vi "DFD Kaiser Order Estimation.vi"(6 "fs [Hz]":dbl=1.0 format="%.2f", 7 "filter type":T3(ring), 8 "error in (no error)":errorcluster, 9 "order option":enum16{"MinNum", "MinEven", "MinOdd"}(ring)=enum."MinEven", 10 "ripple specs":T1={"passband"=0.1, "stopband"=60.0, "dB/linear? (T: dB)"=TRUE}, 11 "freq specs [Hz]":T2={"fpass 1"=0.2, "fstop 1"=0.3, "fpass 2 "=0.0, "fstop 2"=0.0}) -> (0 "error out":errorcluster, 1 "low cutoff freq [Hz]":dbl, 2 "high cutoff freq [Hz]":dbl, 3 "estimated order":i32, 4 "beta":dbl format="%.2f")   [LabVIEW 2017, in "NI_DigFilterLicensed.lvlib"]
doc: "Estimates the order of a finite impulse response (FIR) filter that you designed by using the Kaiser Window method."
uses:
  <vilib>/addons/Digital Filter Design/NI_DigFilterLicensed.lvlib
  <vilib>/addons/Digital Filter Design/_Objects.llb/DFD Filter Frequence Specification (Design).ctl
  <vilib>/addons/Digital Filter Design/_Objects.llb/DFD Filter Ripple Specification (Design).ctl
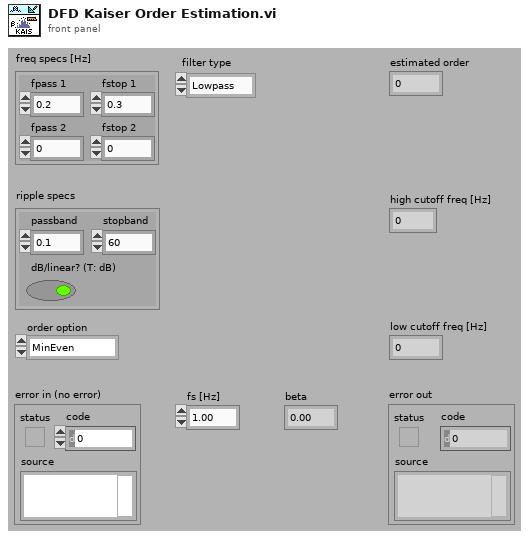
[diagram p1: front panel]
types:
  T1 = typedef "NI_DigFilterLicensed.lvlib/DFD Filter Ripple Specification (Design).ctl" = cluster{"passband":dbl, "stopband":dbl, "dB/linear? (T: dB)":bool}
  T2 = typedef "NI_DigFilterLicensed.lvlib/DFD Filter Frequence Specification (Design).ctl" = cluster{"fpass 1":dbl, "fstop 1":dbl, "fpass 2 ":dbl, "fstop 2":dbl}
  T3 = enum16{"Lowpass", "Highpass", "Bandpass", "Bandstop"}
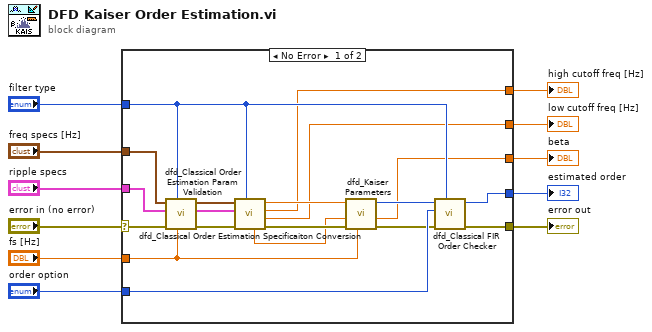
[diagram p0: block diagram]
diagram:
  n1 = case shown="No Error" "error in (no error)" {
    selector: "error in (no error)" -> [w12 w31]
    tunnel: [w30 w31] -> w11
    tunnel: "order option" -> [w29 _]
    tunnel: [w28 _] -> w9
    tunnel: "filter type" -> [w27 _]
    tunnel: "fs [Hz]" -> [w26 _]
    tunnel: "ripple specs" -> [w25 _]
    tunnel: "freq specs [Hz]" -> [w20 _]
    tunnel: [w16 _] -> w4
    tunnel: [w14 _] -> w3
    tunnel: [w13 _] -> w2
    frame No Error {
      n2 = call <vilib>:"dfd_Classical Order Estimation Param Validation.vi"("fs [Hz]"=w26, "filter type"=w27, "error in (no error)"=w12, "ripple specs"=w25, "freq specs [Hz]"=w20) -> ("error out"=w17:errorcluster, "dup ripple specs"=w19:T1, "dup freq specs [Hz]"=w18:T2)  [unwired: 1 in, 3 out]
      n3 = call <vilib>:"dfd_Classical Order Estimation Specificaiton Conversion.vi"("filter type"=w27, "error in (no error)"=w17, "ripple specs"=w19, "freq specs [Hz]"=w18) -> ("error out"=w22:errorcluster, "low cutoff freq: fl"=w13:dbl, "high cutoff freq: fh"=w14:dbl, "min transition band"=w23:dbl, "A stop (dB)"=w15:dbl)  [unwired: 1 in, 2 out]
      n4 = call <vilib>:"dfd_Kaiser Parameters.vi"("fs [Hz]"=w26, "error in (no error)"=w22, "A stop [dB]"=w15, "delta f [Hz]"=w23) -> ("error out"=w21:errorcluster, "beta"=w16:dbl, "order"=w24:i32)  [unwired: 1 in, 4 out]
      n5 = call <vilib>:"dfd_Classical FIR Order Checker.vi"("filter type"=w27, "error in (no error)"=w21, "order option"=w29, "order in"=w24) -> ("error out"=w30:errorcluster, "order out"=w28:i32)  [unwired: 6 out]
    }
    frame Error {
    }
  }
  "error out" <- w11
  "estimated order" <- w9
  "beta" <- w4
  "high cutoff freq [Hz]" <- w3
  "low cutoff freq [Hz]" <- w2
